vi "LaserGain.vi"(7 "LVWSR":refnum<class "Web Request.lvclass">, 9 "B1":dbl, 10 "B0":dbl, 11 "R":dbl) -> ()   [LabVIEW 2014]
uses:
  <vilib>/wsapi/Web Request.lvclass
  Instr Actor/Messages/Change CRD Laser Gain/Change Laser Gain MSG.lvclass
  Controller/Controls/Enqueuer Enum.ctl
  Instr Actor/Messages/Change CRD Laser Gain/Change Laser Gain MSG.lvclass/Change Laser Gain MSG.ctl
  Controller/Controller.lvclass
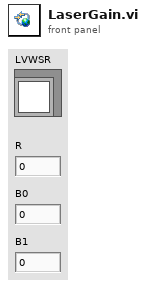
[diagram p1: front panel]
types:
  T1 = typedef "Enqueuer Enum.ctl" = enum8{"PAS", "CRDS", "File"}
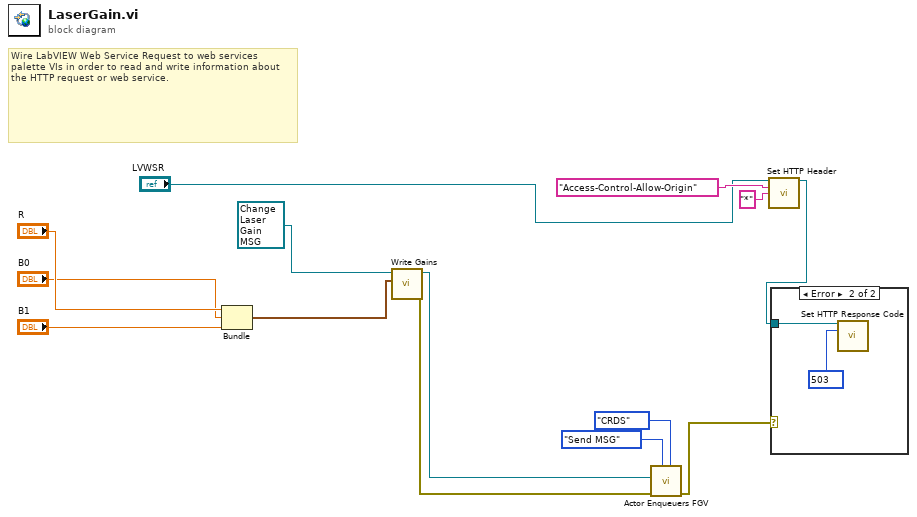
[diagram p0: block diagram]
diagram:
  # "Wire LabVIEW Web Service Request to web services palette VIs in order to read and write information about the HTTP request or web service."
  n1 = Bundle("R"="R", "B0"="B0", "B1"="B1") -> (w11:cluster{"R":dbl, "B0":dbl, "B1":dbl})  [unwired: 1 in]
  n2 = call "Write Gains.vi"("Gains"=w11, "Change Laser Gain MSG in"=refnum<class "Change Laser Gain MSG.lvclass"> refnum ("Instrument Lib:Change Laser Gain MSG")) -> ("error out"=w5:errorcluster, "Change Laser Gain MSG out"=w6:refnum<class "Change Laser Gain MSG.lvclass">)  [unwired: 8 in]
  n3 = call "Actor Enqueuers FGV.vi"("Enqueuer"=Enqueuer_Enum."CRDS", "State"=enum16{"Store", "Send MSG"}."Send MSG", "error in"=w5, "MSG"=w6) -> ("error out"=w9:errorcluster)  [unwired: 7 in]
  n4 = call <vilib>:"Set HTTP Header.vi"("LabVIEW Web Service Request"="LVWSR", "header"="Access-Control-Allow-Origin", "header value"="*") -> ("LabVIEW Web Service Request out"=w1:refnum<class "Web Request.lvclass">)  [unwired: 11 in, 1 out]
  n5 = case shown="Error" w9 {
    tunnel: w1 -> [_ w16]
    frame No Error {
    }
    frame Error {
      w15 = 503 items=["100"=100, "101"=101, "200"=200, "201"=201, "202"=202, "203"=203, "204"=204, "205"=205, "206"=206, "300"=300, "301"=301, "302"=302, "303"=303, "304"=304, "305"=305, "306"=306, "307"=307, "400"=400, "401"=401, "402"=402, "403"=403, "404"=404, "405"=405, "406"=406, "407"=407, "408"=408, "409"=409, "410"=410, "411"=411, "412"=412, "413"=413, "414"=414, "415"=415, "416"=416, "417"=417, "500"=500, "501"=501, "502"=502, "503"=503, "504"=504, "505"=505] ("response code (200)")
      n6 = call <vilib>:"Set HTTP Response Code.vi"("LabVIEW Web Service Request"=w16, "response code (200)"=w15) -> ()  [unwired: 12 in, 2 out]
    }
  }
